vi "variantCtrlBoolean.vi"(4 "isRequired (T)":bool=TRUE, 6 "menu in (get)":enum16{"get", "set"}(ring), 8 "error in":errorcluster, 9 "Boolean Value in":bool, 10 "name in":string, 11 "variant in":variant) -> (0 "error out":errorcluster, 1 "Boolean Value out":bool, 2 "isFound?":bool, 3 "variant out":variant)   [LabVIEW 2024]
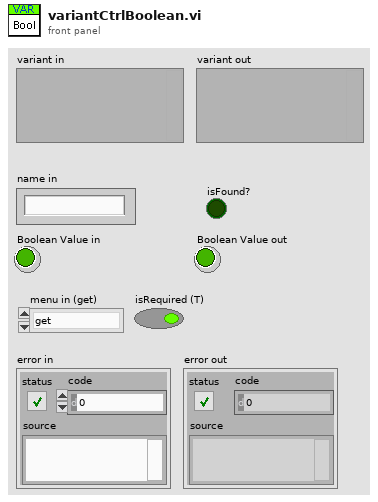
[diagram p1: front panel]
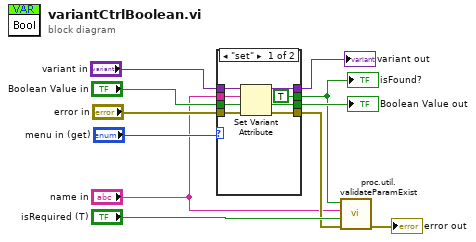
[diagram p0: block diagram]
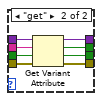
[diagram p2: hidden frame]
diagram:
  n1 = case shown="\"set\"" "menu in (get)" {
    tunnel: "error in" -> [w18 w26]
    tunnel: "Boolean Value in" -> [w13 w25]
    tunnel: "variant in" -> [w17 w24]
    tunnel: [w16 w23] -> w3
    tunnel: [TRUE w22] -> w4
    tunnel: [w15 w21] -> w8
    tunnel: "name in" -> [w14 w20]
    tunnel: [w13 w19] -> w6
    frame "set" {
      n2 = Set Variant Attribute(Variant=w17, name=w14, value=w13, error in=w18) -> (Variant out=w15:variant, error out=w16:errorcluster)  [unwired: 1 out]
    }
    frame "get" {
      n3 = Get Variant Attribute(Variant=w24, name=w20, default value (empty Variant)=w25, error in=w26) -> (duplicate Variant=w21:variant, found=w22:bool, value=w19:bool, error out=w23:errorcluster)
    }
  }
  "isFound?" <- w4
  "variant out" <- w8
  "Boolean Value out" <- w6
  n4 = call "proc.util.validateParamExist.vi"("error in"=w3, "isRequired"="isRequired (T)", "Param Label"="name in", "isFound"=w4) -> ("error out"=→"error out":errorcluster)  [unwired: 7 in]
